vi "GlobalLaserInterface.vi"() -> ()   [LabVIEW 2010]
panel:
  in  "InterfaceLaserInitalised":refnum<visa-resource-name>
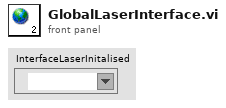
[diagram p1: front panel]
diagram:
